vi "CRYGet Active Graph Ref to DVIndex.vi"(11 "DV Array index":i32) -> (0 "Title State":bool, 1 "Frame VIRef":refnum<vi>, 2 "sQueueName":string, 3 "Inserted Graph VIRef out":refnum<vi>, 4 "Graph Main VIRef":refnum<vi>, 5 "Graph VIRef Array Index":i32=-1)   [LabVIEW 2013]
uses:
  CRYNew View Global.vi
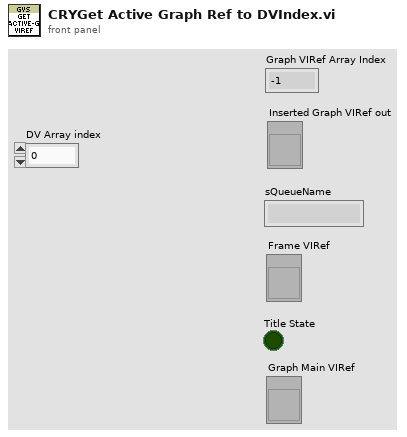
[diagram p1: front panel]
types:
  T1 = typedef "Graph Main Info Cluster.ctl" = cluster{"Selected_BarIdx":i32, "Selected_PanelIdx":i32, "Graph Main VIRef":refnum<vi>, "ToolBarClick":bool, "Spliter Ref Array":refnum<vi>[], "Panel Ref Array":refnum<vi>[], "Spliter_matrix":i32[][], "Panel_matrix":i32[][], "child_spliterIdx_matrix":i32[][], "split_pos_matrix":i32[][], "Title State":bool, "sQueueName":string, "Frame nID":i32, "Graph VIRef Array":cluster{"Graph VIRef":refnum<vi>, "Panel Idx":i32, "Frame VIRef":refnum<vi>, "Icon Ring":i32, "Graph Type":string}[], "View Type":string}
  T2 = cluster{"Graph VIRef":refnum<vi>, "Panel Idx":i32, "Frame VIRef":refnum<vi>, "Icon Ring":i32, "Graph Type":string}[]
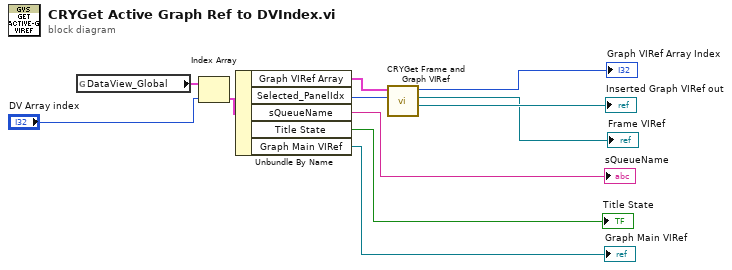
[diagram p0: block diagram]
diagram:
  n1 = global read "CRYNew View Global.vi" "DataView_Global"() -> (w4:T1[])
  n2 = Index Array(array=w4, index="DV Array index") -> (element=w11:T1)
  n3 = Unbundle By Name(w11) -> ("Graph VIRef Array"=w7:T2, "Selected_PanelIdx"=w8:i32, "sQueueName"=→"sQueueName":string, "Title State"=→"Title State":bool, "Graph Main VIRef"=→"Graph Main VIRef":refnum<vi>)
  n4 = call "CRYGet Frame and Graph VIRef.vi"("Panel Idx"=w8, "Graph VIRef Array"=w7) -> ("Graph VIRef"=→"Inserted Graph VIRef out":refnum<vi>, "Frame VIRef"=→"Frame VIRef":refnum<vi>, "Graph VIRef Array Index"=→"Graph VIRef Array Index":i32)  [unwired: 5 in, 2 out]
